vi "Update Test Information.vi"(8 "error in":errorcluster, 11 "Test Information":T1={"APU Part Number:"="", "Model:"="", "Serial Number:"="", "Customer:"="", "Work Order:"="", "Pre or Post SB"="", "Run Count"=0, "APU Selected"="<Select>"} {"Run Count" min=0 step=1}) -> (0 "error out":errorcluster)   [LabVIEW 2018, in "Controller (Host).lvlib"]
doc: "This subVI enqueues the named action in to the communications queue along with the input data."
uses:
  Controller (Host).lvlib
  Public Controls/Test Information.ctl
  Public VIs/PreorPostSB.ctl
  Public Controls/APU Select.ctl
  Private Controls/Module Data.ctl
  Private Controls/Module Action.ctl
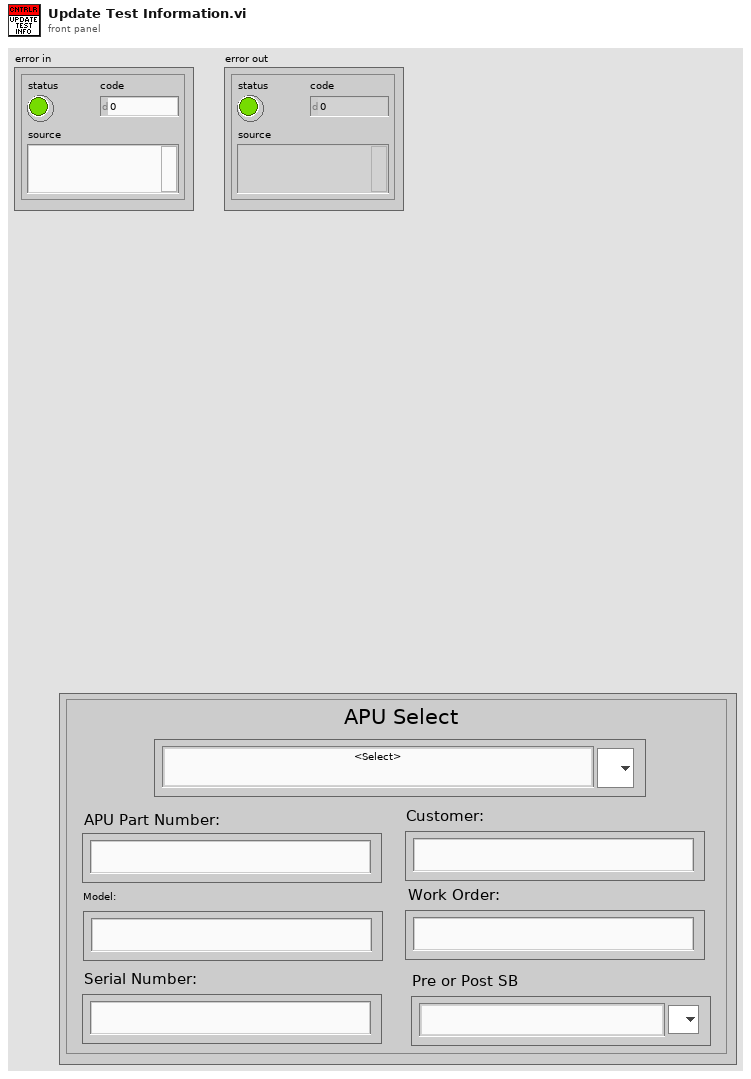
[diagram p1: front panel]
types:
  T1 = typedef "Controller (Host).lvlib/Test Information.ctl" = cluster{"APU Part Number:":string, "Model:":string, "Serial Number:":string, "Customer:":string, "Work Order:":string, "Pre or Post SB":T2, "Run Count":i32, "APU Selected":T3}
  T2 = typedef "Controller (Host).lvlib/PreorPostSB.ctl" = string
  T3 = typedef "Controller (Host).lvlib/APU Select.ctl" = string
  T4 = typedef "Controller (Host).lvlib/Module Data.ctl" = cluster{"Data":variant, "Action":T5}
  T5 = typedef "Controller (Host).lvlib/Module Action.ctl" = enum8{"Timeout", "New Data", "Value to Monitor", "Init", "Reset Dev_Min_Max", "Error", "Exit", "Prompt Test Info", "Update Test Info", "Prompt Variable Info", "Load APU Setup Data"}
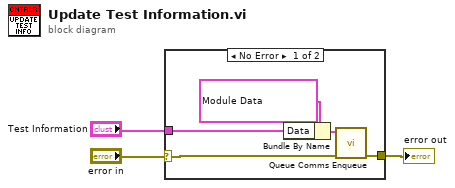
[diagram p0: block diagram]
diagram:
  n1 = case shown="No Error" "error in" {
    selector: "error in" -> [w7 w9]
    tunnel: [w8 w9] -> w3
    tunnel: "Test Information" -> [w4 _]
    frame No Error {
      n2 = Bundle By Name(cluster=T4 {"Data"=variant, "Action"=enum."Update Test Info"} ("Module Data"), "Data"=w4) -> (w5:T4)
      n3 = call "Queue Comms Enqueue.vi"("error in (no error)"=w7, "element"=w5) -> ("error out"=w8:errorcluster)  [unwired: 9 in]
    }
    frame Error {
    }
  }
  "error out" <- w3
